vi "onDestroyHttpSession.vi"(8 "error in (no error)":errorcluster, 11 "REST Client in":refnum<class "REST Client.lvclass">) -> (0 "error out":errorcluster, 3 "REST Client out":refnum<class "REST Client.lvclass">)   [LabVIEW 2020, in "REST Client.lvlib" / "REST Client.lvclass"]
uses:
  REST Client.lvclass
  REST Client.lvclass/REST Client.ctl
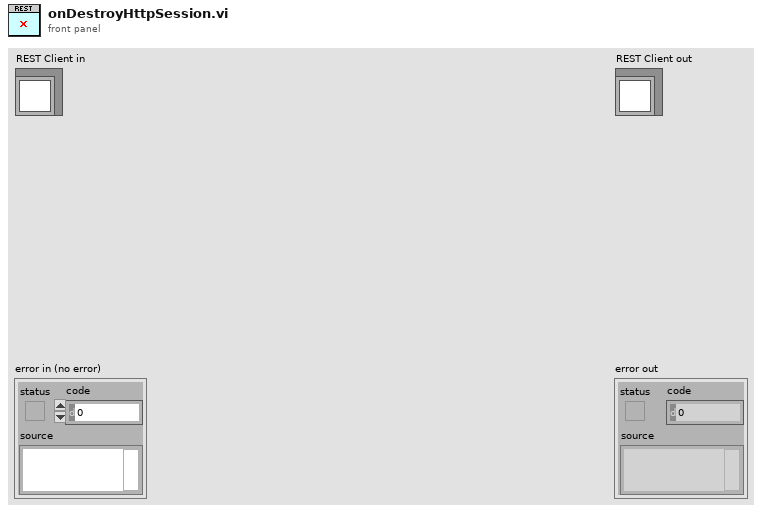
[diagram p1: front panel]
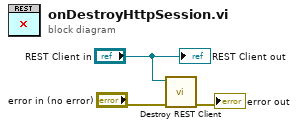
[diagram p0: block diagram]
diagram:
  n1 = call-dynamic "Destroy REST Client.vi"("error in (no error)"="error in (no error)", "REST Client in"="REST Client in") -> ("error out"=→"error out":errorcluster)  [unwired: 9 in]
  "REST Client out" <- "REST Client in"
